vi "DunkFlips.vi"() -> ()   [LabVIEW 2015]
uses:
  <vilib>/eio/EIONode/EIONode.xnode
  <vilib>/rvi/eio/common/nirviEmuTemplateMethod_errors.vi
  <vilib>/rvi/DataTransferAndStorage/Container/XNode/niFpgaContainer.xnode
  <vilib>/rvi/LocalResourceManager/LocalResourceManager.xnode
  <vilib>/rvi/FIFO/Fifo_Resource/niFpgaFifoEmulationRefIn.vi
  <vilib>/rvi/DataTransferAndStorage/Container/Common/niFpgaContainerGetUniqueNameForEmu.vi
  <vilib>/rvi/DataTransferAndStorage/Container/Common/niFpgaContainerSetEmuInfo.vi
  <vilib>/rvi/eio/common/nirviEmuReportErrorAndStop.vi
  <vilib>/rvi/Analysis/measure/period/XNode/niFpgaAnalogPeriod.xnode
  <vilib>/rvi/Analysis/measure/period/templates/niFPGA Period Edge Direction.ctl
  <vilib>/rvi/Analysis/common/codeGenErrors/XNode/niFpgaXNodeCodeGenErrorHandle.vi
  <vilib>/rvi/Analysis/utilities/niFPGA Threshold Crossing Logic.vi
  <vilib>/Platform/TimedLoop/XDataNode/XDataNode.xnode
  <vilib>/Platform/TimedLoop/XDataNode/timing_clust.ctl
  <vilib>/Platform/TimedLoop/XDataNode/XDNodeRunTimeDep.lvlib
  <vilib>/Platform/TimedLoop/XDataNode/wakeup.ctl
  <vilib>/Platform/TimedLoop/XDataNode/nitl_modes.ctl
  <vilib>/rvi/FXPMathLib/basic elements/FxpDiscreteDelay/XNode/nifxpmath_DiscreteDelay.xnode
  <vilib>/rvi/interface/RandomDataEmulation/nirviRandomDataFpgaReadWriteTemplate.vi
  <vilib>/rvi/Analysis/measure/butterworth/XNode/niFpgaButterworthFilter.xnode
panel:
  in  "High Pass":bool
  in  "Low Pass":bool
  in  "Hysteresis 4":fxp<+,8,7> format="%#_13g"
  in  "Hysteresis 3":fxp<+,8,7> format="%#_13g"
  in  "Hysteresis 2":fxp<+,8,7> format="%#_13g"
  out "Actual Sample Period Process (ticks)":u32=80
  in  "Min signal time gap (samples)":u32=1000000
  in  "Min Amplitude 1":fxp<+,16,8>
  out "Output 1":i32
  out "AI0":sgl(slide) scale=-10.0..10.0
  in  "Min Amplitude 2":fxp<+,16,8>
  out "Output 2":i32
  out "AI1":sgl(slide) scale=-10.0..10.0
  in  "Min Amplitude 3":fxp<+,16,8>
  out "Output 3":i32
  out "AI2":sgl(slide) scale=-10.0..10.0
  out "Output 4":i32
  in  "Max Period (samples)":fxp<+,16,16>=65535.0 format="%#_13g"
  in  "Min Period (samples)":fxp<+,16,16> format="%#_13g"
  in  "Hysteresis 1":fxp<+,8,7> format="%#_13g"
  in  "Min Amplitude 4":fxp<+,16,8>
  out "AI3":sgl(slide)=8.326673e-17 scale=-10.0..10.0
  in  "Requested Sample Period (ticks)":u32=80
  out "Invalid Period":bool
  out "Actual Sample Period Wave (ticks)":u32=80
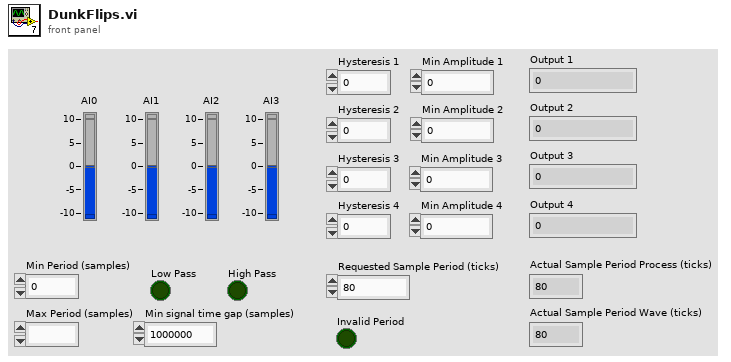
[diagram p1: front panel]
types:
  T1 = typedef "XDNodeRunTimeDep.lvlib/timing_clust.ctl" = cluster{"Expected End [f-1]":u64, "Actual End [f-1]":u64, "Finished Late? [f-1]":bool, "Expected End [i-1]":u64, "Actual End [i-1]":u64, "Finished Late? [i-1]":bool, "Expected Start [i]":u64, "Actual Start [i]":u64, "Expected Start [f]":u64, "Actual Start [f]":u64, "Source Name":string, "Structure Name":string, "Period":i64, "Deadline":i64, "Offset":i64, "Start":i64, "Priority":i32, "Timeout":i32, "Mode":T2, "Wakeup Reason":T3, "Error":errorcluster, "Source Type":string, "Secondary Source Type":string, "Global End Time":u64, "Global Start Time":u64, "Frame Duration":u64, "Iteration Duration":u64, "Assigned CPU":i32, "I/O Scan Engine Mode":u32}
  T2 = typedef "XDNodeRunTimeDep.lvlib/nitl_modes.ctl" = enum32{"No Change", "Process missed periods, maintain original phase", "Discard missed periods, maintain original phase", "Process missed periods, ignore original phase", "Discard missed periods, ignore original phase"}
  T3 = typedef "XDNodeRunTimeDep.lvlib/wakeup.ctl" = enum32{"Normal", "Aborted", "Asynchronous wakeup", "Timing source error", "Timed loop error", "Timeout"}
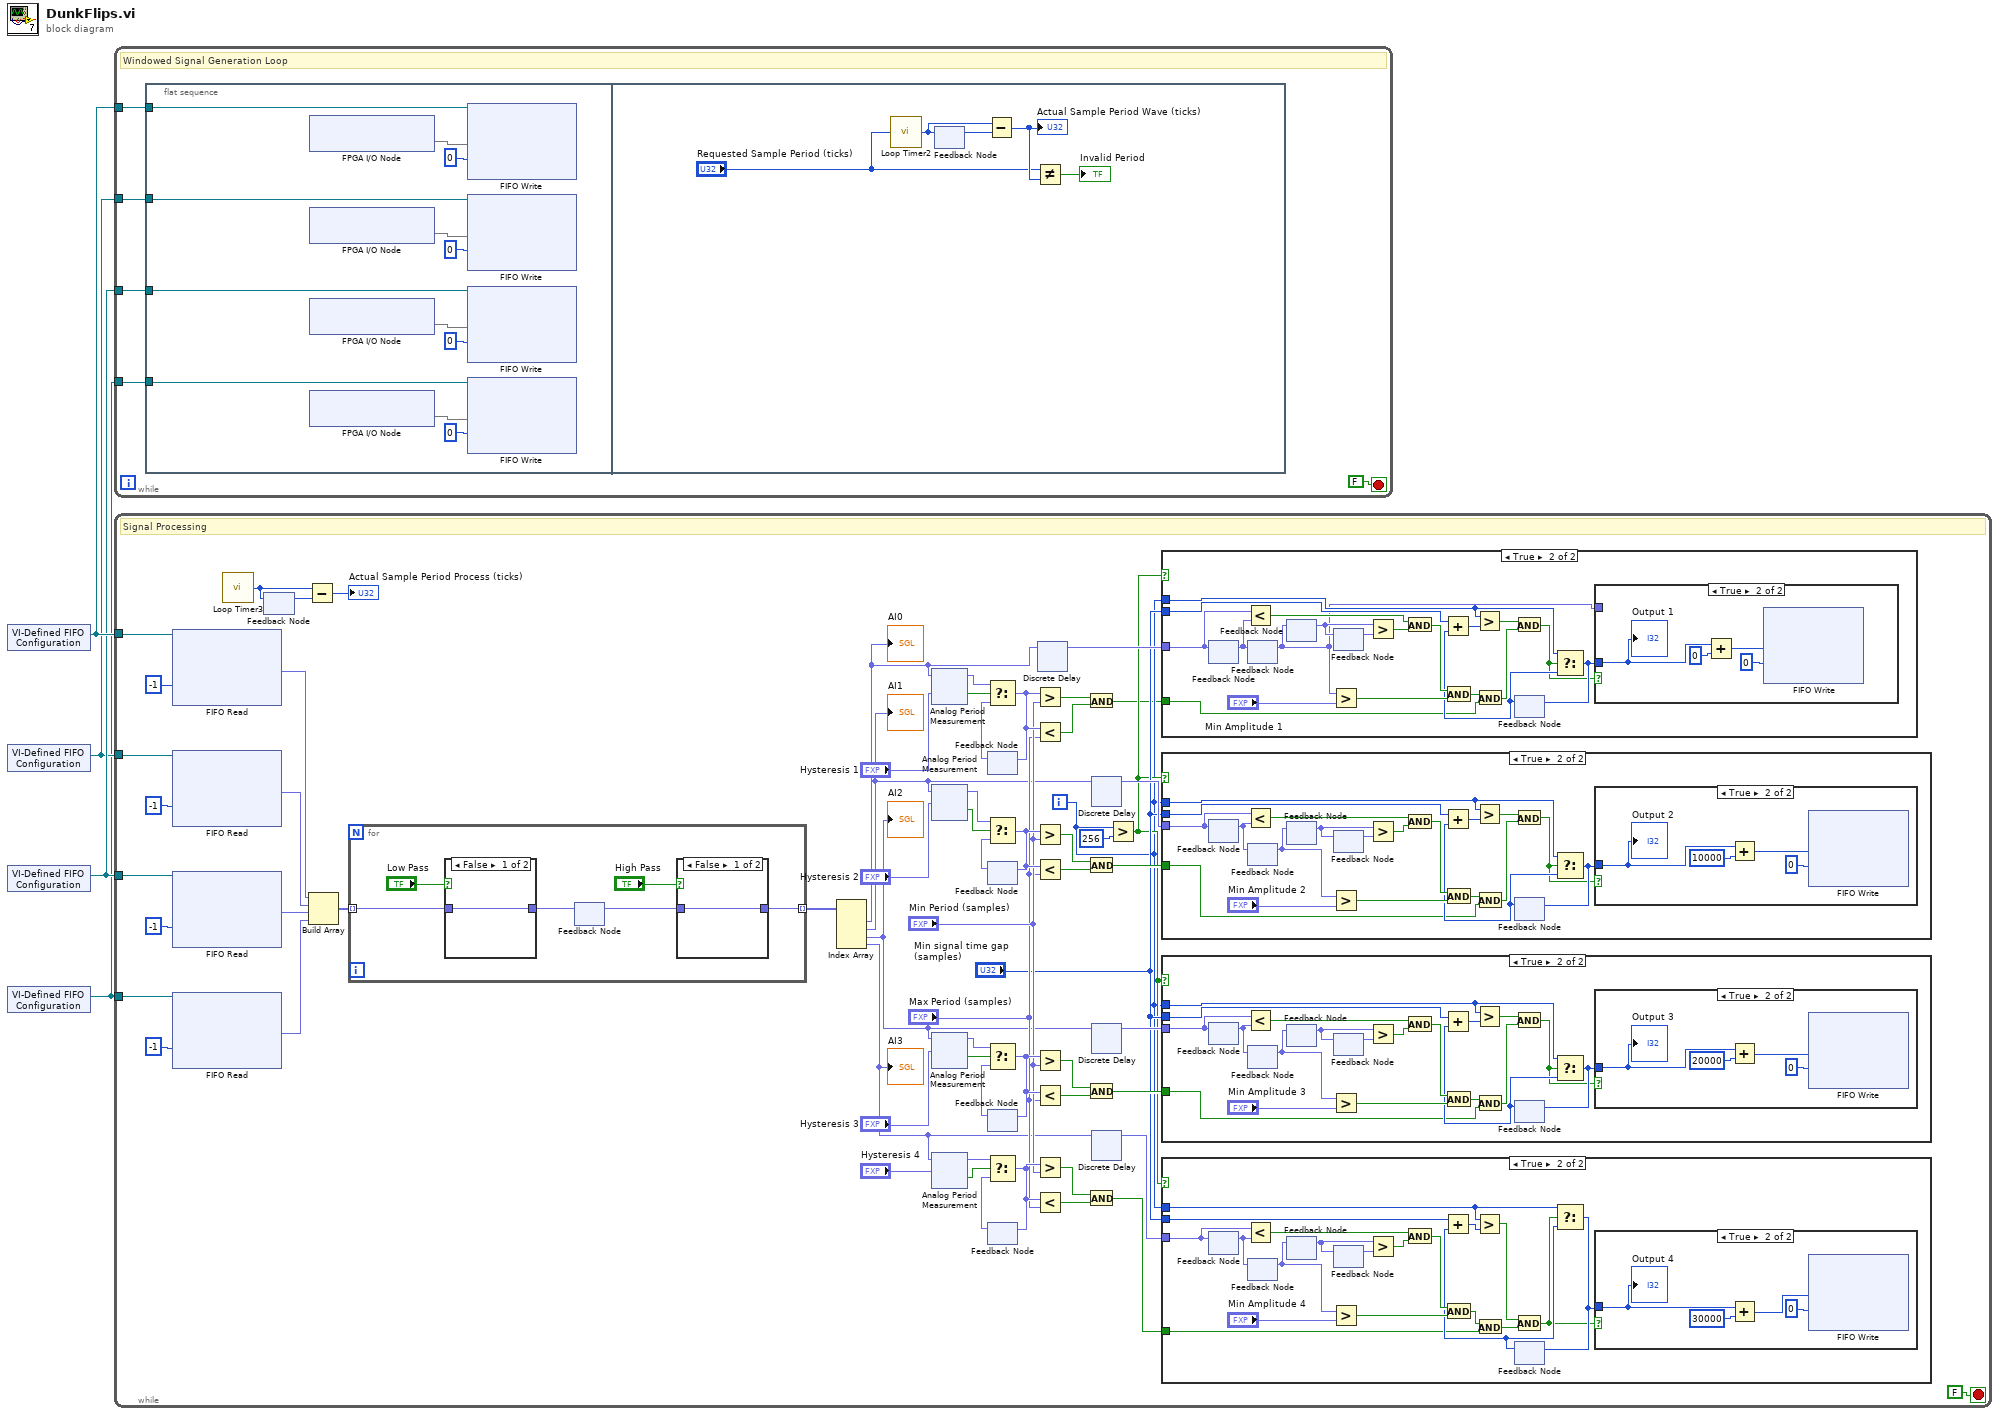
[diagram p0: block diagram]
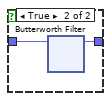
[diagram p2: hidden frame]
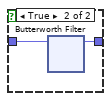
[diagram p3: hidden frame]
diagram:
  n1 = xnode "VI-Defined FIFO Configuration"() -> ("FIFO Out"=w4:refnum<k21>)
  n2 = xnode "VI-Defined FIFO Configuration"() -> ("FIFO Out"=w2:refnum<k21>)
  n3 = xnode "VI-Defined FIFO Configuration"() -> ("FIFO Out"=w3:refnum<k21>)
  n4 = xnode "VI-Defined FIFO Configuration"() -> ("FIFO Out"=w1:refnum<k21>)
  n5 = while {
    tunnel: w4 -> [w9]
    tunnel: w2 -> [w7]
    tunnel: w3 -> [w6]
    tunnel: w1 -> [w5]
    stop <- FALSE stop-if-true
    # "Windowed Signal Generation Loop"
    n6 = flat-sequence {
      tunnel: w9 -> [w16]
      tunnel: w7 -> [w15]
      tunnel: w6 -> [w14]
      tunnel: w5 -> [w17]
      frame #0 {
        n7 = xnode "FPGA I/O Node"() -> ("Connector0/AI0"=w13)  [unwired: 1 in, 1 out]
        n8 = xnode "FPGA I/O Node"() -> ("Connector0/AI1"=w10)  [unwired: 1 in, 1 out]
        n9 = xnode "FPGA I/O Node"() -> ("Connector0/AI2"=w11)  [unwired: 1 in, 1 out]
        n10 = xnode "FPGA I/O Node"() -> ("Connector0/AI3"=w12)  [unwired: 1 in, 1 out]
        n11 = xnode ("FIFO Write")("Element"=w13, "Timeout"=0, "FIFO In"=w16) -> ()  [unwired: 2 out]
        n12 = xnode ("FIFO Write")("Element"=w10, "Timeout"=0, "FIFO In"=w15) -> ()  [unwired: 2 out]
        n13 = xnode ("FIFO Write")("Element"=w11, "Timeout"=0, "FIFO In"=w14) -> ()  [unwired: 2 out]
        n14 = xnode ("FIFO Write")("Element"=w12, "Timeout"=0, "FIFO In"=w17) -> ()  [unwired: 2 out]
      }
      frame #1 {
        n15 = call "Loop Timer2"("Count(Ticks)"="Requested Sample Period (ticks)") -> ("Tick Count(Ticks)"=w22:u32)
        n16 = feedback #1() -> (w23:u32)  [unwired: 1 in]
        n17 = feedback-in #1(w22) -> ()
        n18 = Subtract(x=w22, y=w23) -> (x-y=w26:u32)
        "Actual Sample Period Wave (ticks)" <- w26
        n19 = Not Equal?(x="Requested Sample Period (ticks)", y=w26) -> (x != y?=→"Invalid Period":bool)
      }
    }
  }
  n20 = while {
    tunnel: w4 -> [w60]
    tunnel: w2 -> [w61]
    tunnel: w3 -> [w59]
    tunnel: w1 -> [w81]
    i -> [w50]
    stop <- FALSE stop-if-true
    # "Signal Processing"
    n21 = xnode ("FIFO Read")("Timeout"=i16 -1, "FIFO In"=w60) -> ("Element"=w30:fxp<+/-,16,4>)  [unwired: 2 out]
    n22 = xnode ("FIFO Read")("Timeout"=i16 -1, "FIFO In"=w61) -> ("Element"=w29:fxp<+/-,16,4>)  [unwired: 2 out]
    n23 = xnode ("FIFO Read")("Timeout"=i16 -1, "FIFO In"=w59) -> ("Element"=w28:fxp<+/-,16,4>)  [unwired: 2 out]
    n24 = xnode ("FIFO Read")("Timeout"=i16 -1, "FIFO In"=w81) -> ("Element"=w27:fxp<+/-,16,4>)  [unwired: 2 out]
    n25 = call "Loop Timer3"() -> ("Tick Count(Ticks)"=w51:u32)  [unwired: 1 in]
    n26 = feedback #2() -> (w52:u32)  [unwired: 1 in]
    n27 = feedback-in #2(w51) -> ()
    n28 = Subtract(x=w51, y=w52) -> (x-y=→"Actual Sample Period Process (ticks)":u32)
    n29 = Build Array(w30, w29, w28, w27) -> (w36:fxp<+/-,16,4>[])
    n30 = for {
      tunnel: w36 -> [w93] mode=indexing
      tunnel: [w94] -> w35 mode=indexing
      n31 = case shown="False" "Low Pass" {
        tunnel: [w109 w111] -> w96
        tunnel: w93 -> [w109 w110]
        frame False {
        }
        frame True {
          n32 = xnode "Butterworth Filter"("input data"=w110) -> ("output data"=w111:fxp<+/-,20,8>)  [unwired: 2 in, 1 out]
        }
      }
      n33 = feedback #3() -> (w95:fxp<+/-,20,8>)  [unwired: 1 in]
      n34 = feedback-in #3(w96) -> ()
      n35 = case shown="False" "High Pass" {
        tunnel: w95 -> [w97 w99]
        tunnel: [w97 w98] -> w94
        frame False {
        }
        frame True {
          n36 = xnode "Butterworth Filter"("input data"=w99) -> ("output data"=w98:fxp<+/-,20,12>)  [unwired: 2 in, 1 out]
        }
      }
    }
    n37 = Index Array(array=w35) -> (element #1=w34:fxp<+/-,24,12>, element #2=w33:fxp<+/-,24,12>, element #3=w32:fxp<+/-,24,12>, element #4=w31:fxp<+/-,24,12>)  [unwired: 4 in]
    "AI3" <- w31
    "AI2" <- w32
    "AI1" <- w33
    "AI0" <- w34
    n38 = xnode "Analog Period Measurement"("input data"=w34, "direction"="Hysteresis 1") -> ("period (samples)"=w48:fxp<+,32,16>, "output valid"=w64:bool)  [unwired: 3 in, 2 out]
    n39 = xnode "Analog Period Measurement"("input data"=w33, "hysteresis"="Hysteresis 2") -> ("period (samples)"=w46:fxp<+,32,16>, "output valid"=w69:bool)  [unwired: 3 in, 2 out]
    n40 = xnode "Analog Period Measurement"("input data"=w32, "hysteresis"="Hysteresis 3") -> ("period (samples)"=w44:fxp<+,32,16>, "output valid"=w75:bool)  [unwired: 3 in, 2 out]
    n41 = xnode "Analog Period Measurement"("input data"=w31, "hysteresis"="Hysteresis 4") -> ("period (samples)"=w42:fxp<+,32,16>, "output valid"=w83:bool)  [unwired: 3 in, 2 out]
    n42 = feedback #4() -> (w47:fxp<+,32,16>)  [unwired: 1 in]
    n43 = Select(t=w48, s=w64, f=w47) -> (s? t:f=w66:fxp<+,32,16>)
    n44 = feedback-in #4(w66) -> ()
    n45 = feedback #5() -> (w45:fxp<+,32,16>)  [unwired: 1 in]
    n46 = Select(t=w46, s=w69, f=w45) -> (s? t:f=w71:fxp<+,32,16>)
    n47 = feedback-in #5(w71) -> ()
    n48 = feedback #6() -> (w43:fxp<+,32,16>)  [unwired: 1 in]
    n49 = Select(t=w44, s=w75, f=w43) -> (s? t:f=w77:fxp<+,32,16>)
    n50 = feedback-in #6(w77) -> ()
    n51 = feedback #7() -> (w41:fxp<+,32,16>)  [unwired: 1 in]
    n52 = Select(t=w42, s=w83, f=w41) -> (s? t:f=w86:fxp<+,32,16>)
    n53 = feedback-in #7(w86) -> ()
    n54 = Greater?(x=w66, y="Min Period (samples)") -> (0:w68:bool)
    n55 = Less?(x=w66, y="Max Period (samples)") -> (x < y?=w67:bool)
    n56 = Greater?(x=w71, y="Min Period (samples)") -> (0:w73:bool)
    n57 = Less?(x=w71, y="Max Period (samples)") -> (x < y?=w72:bool)
    n58 = Greater?(x=w77, y="Min Period (samples)") -> (0:w79:bool)
    n59 = Less?(x=w77, y="Max Period (samples)") -> (x < y?=w78:bool)
    n60 = Greater?(x=w86, y="Min Period (samples)") -> (0:w88:bool)
    n61 = Less?(x=w86, y="Max Period (samples)") -> (x < y?=w87:bool)
    n62 = xnode ("Discrete Delay")("D"=w34) -> ("Q"=w65:fxp<+/-,24,12>)
    n63 = And(x=w68, y=w67) -> (x .and. y?=w49:bool)
    n64 = And(x=w73, y=w72) -> (x .and. y?=w74:bool)
    n65 = And(x=w79, y=w78) -> (x .and. y?=w80:bool)
    n66 = And(x=w88, y=w87) -> (x .and. y?=w89:bool)
    n67 = xnode ("Discrete Delay")("D"=w33) -> ("Q"=w70:fxp<+/-,24,12>)
    n68 = xnode ("Discrete Delay")("D"=w32) -> ("Q"=w76:fxp<+/-,24,12>)
    n69 = xnode ("Discrete Delay")("D"=w31) -> ("Q"=w84:fxp<+/-,24,12>)
    n70 = Greater?(x=w50, y=i16 256) -> (0:w57:bool)
    n71 = case shown="True" w57 {
      tunnel: w50 -> [_ w134]
      tunnel: w65 -> [_ w130]
      tunnel: w49 -> [_ w126]
      tunnel: "Min signal time gap (samples)" -> [_ w125]
      frame False {
      }
      frame True {
        n72 = feedback #8() -> (w138:fxp<+/-,24,12>)  [unwired: 1 in]
        n73 = feedback-in #8(w130) -> ()
        n74 = Less?(x=w130, y=w138) -> (x < y?=w122:bool)
        n75 = feedback #9() -> (w121:fxp<+/-,24,12>)  [unwired: 1 in]
        n76 = feedback-in #9(w138) -> ()
        n77 = feedback #10() -> (w139:fxp<+/-,24,12>)  [unwired: 1 in]
        n78 = feedback-in #10(w121) -> ()
        n79 = Greater?(x=w121, y="Min Amplitude 1") -> (0:w133:bool)
        n80 = feedback #11() -> (w140:fxp<+/-,24,12>)  [unwired: 1 in]
        n81 = feedback-in #11(w139) -> ()
        n82 = Greater?(x=w139, y=w140) -> (0:w123:bool)
        n83 = And(x=w122, y=w123) -> (x .and. y?=w135:bool)
        n84 = And(x=w135, y=w133) -> (x .and. y?=w128:bool)
        n85 = And(x=w128, y=w126) -> (x .and. y?=w127:bool)
        n86 = feedback #12() -> (w131:i32)  [unwired: 1 in]
        n87 = Add(x=w125, y=w131) -> (x+y=w137:u32)
        n88 = Greater?(x=w134, y=w137) -> (0:w124:bool)
        n89 = And(x=w124, y=w127) -> (x .and. y?=w129:bool)
        n90 = Select(t=w134, s=w129, f=w131) -> (s? t:f=w132:i32)
        n91 = feedback-in #12(w132) -> ()
        n92 = case shown="True" w129 {
          tunnel: w132 -> [_ w142]
          tunnel: w121 -> [_ _]
          frame False {
          }
          frame True {
            n93 = Add(x=w142, y=i16 0) -> (x+y=w141:i32)
            n94 = xnode ("FIFO Write")("Element"=w141, "Timeout"=i16 0) -> ()  [unwired: 1 in, 2 out]
            "Output 1" <- w142
          }
        }
      }
    }
    n95 = case shown="True" w57 {
      tunnel: w50 -> [_ w274]
      tunnel: w70 -> [_ w269]
      tunnel: w74 -> [_ w265]
      tunnel: "Min signal time gap (samples)" -> [_ w264]
      frame False {
      }
      frame True {
        n96 = feedback #13() -> (w279:fxp<+/-,24,12>)  [unwired: 1 in]
        n97 = feedback-in #13(w269) -> ()
        n98 = Less?(x=w269, y=w279) -> (x < y?=w263:bool)
        n99 = feedback #14() -> (w277:fxp<+/-,24,12>)  [unwired: 1 in]
        n100 = feedback-in #14(w279) -> ()
        n101 = feedback #15() -> (w280:fxp<+/-,24,12>)  [unwired: 1 in]
        n102 = feedback-in #15(w277) -> ()
        n103 = Greater?(x=w277, y="Min Amplitude 2") -> (0:w272:bool)
        n104 = feedback #16() -> (w281:fxp<+/-,24,12>)  [unwired: 1 in]
        n105 = feedback-in #16(w280) -> ()
        n106 = Greater?(x=w280, y=w281) -> (0:w262:bool)
        n107 = And(x=w263, y=w262) -> (x .and. y?=w275:bool)
        n108 = And(x=w275, y=w272) -> (x .and. y?=w267:bool)
        n109 = And(x=w267, y=w265) -> (x .and. y?=w266:bool)
        n110 = feedback #17() -> (w270:i32)  [unwired: 1 in]
        n111 = Add(x=w264, y=w270) -> (x+y=w278:u32)
        n112 = Greater?(x=w274, y=w278) -> (0:w273:bool)
        n113 = And(x=w273, y=w266) -> (x .and. y?=w268:bool)
        n114 = Select(t=w274, s=w268, f=w270) -> (s? t:f=w271:i32)
        n115 = feedback-in #17(w271) -> ()
        n116 = case shown="True" w268 {
          tunnel: w271 -> [_ w283]
          frame False {
          }
          frame True {
            n117 = Add(x=w283, y=i16 10000) -> (x+y=w282:i32)
            n118 = xnode ("FIFO Write")("Element"=w282, "Timeout"=i16 0) -> ()  [unwired: 1 in, 2 out]
            "Output 2" <- w283
          }
        }
      }
    }
    n119 = case shown="True" w57 {
      tunnel: w50 -> [_ w415]
      tunnel: w76 -> [_ w410]
      tunnel: w80 -> [_ w406]
      tunnel: "Min signal time gap (samples)" -> [_ w405]
      frame False {
      }
      frame True {
        n120 = feedback #18() -> (w420:fxp<+/-,24,12>)  [unwired: 1 in]
        n121 = feedback-in #18(w410) -> ()
        n122 = Less?(x=w410, y=w420) -> (x < y?=w403:bool)
        n123 = feedback #19() -> (w418:fxp<+/-,24,12>)  [unwired: 1 in]
        n124 = feedback-in #19(w420) -> ()
        n125 = feedback #20() -> (w421:fxp<+/-,24,12>)  [unwired: 1 in]
        n126 = feedback-in #20(w418) -> ()
        n127 = Greater?(x=w418, y="Min Amplitude 3") -> (0:w413:bool)
        n128 = feedback #21() -> (w422:fxp<+/-,24,12>)  [unwired: 1 in]
        n129 = feedback-in #21(w421) -> ()
        n130 = Greater?(x=w421, y=w422) -> (0:w404:bool)
        n131 = And(x=w403, y=w404) -> (x .and. y?=w416:bool)
        n132 = And(x=w416, y=w413) -> (x .and. y?=w408:bool)
        n133 = And(x=w408, y=w406) -> (x .and. y?=w407:bool)
        n134 = feedback #22() -> (w411:i32)  [unwired: 1 in]
        n135 = Add(x=w405, y=w411) -> (x+y=w419:u32)
        n136 = Greater?(x=w415, y=w419) -> (0:w414:bool)
        n137 = And(x=w414, y=w407) -> (x .and. y?=w409:bool)
        n138 = Select(t=w415, s=w409, f=w411) -> (s? t:f=w412:i32)
        n139 = feedback-in #22(w412) -> ()
        n140 = case shown="True" w409 {
          tunnel: w412 -> [_ w424]
          frame False {
          }
          frame True {
            n141 = Add(x=w424, y=i16 20000) -> (x+y=w423:i32)
            n142 = xnode ("FIFO Write")("Element"=w423, "Timeout"=i16 0) -> ()  [unwired: 1 in, 2 out]
            "Output 3" <- w424
          }
        }
      }
    }
    n143 = case shown="True" w57 {
      tunnel: w50 -> [_ w556]
      tunnel: w84 -> [_ w551]
      tunnel: w89 -> [_ w547]
      tunnel: "Min signal time gap (samples)" -> [_ w546]
      frame False {
      }
      frame True {
        n144 = feedback #23() -> (w561:fxp<+/-,24,12>)  [unwired: 1 in]
        n145 = feedback-in #23(w551) -> ()
        n146 = Less?(x=w551, y=w561) -> (x < y?=w544:bool)
        n147 = feedback #24() -> (w559:fxp<+/-,24,12>)  [unwired: 1 in]
        n148 = feedback-in #24(w561) -> ()
        n149 = feedback #25() -> (w562:fxp<+/-,24,12>)  [unwired: 1 in]
        n150 = feedback-in #25(w559) -> ()
        n151 = Greater?(x=w559, y="Min Amplitude 4") -> (0:w554:bool)
        n152 = feedback #26() -> (w563:fxp<+/-,24,12>)  [unwired: 1 in]
        n153 = feedback-in #26(w562) -> ()
        n154 = Greater?(x=w562, y=w563) -> (0:w545:bool)
        n155 = And(x=w544, y=w545) -> (x .and. y?=w557:bool)
        n156 = And(x=w557, y=w554) -> (x .and. y?=w549:bool)
        n157 = And(x=w549, y=w547) -> (x .and. y?=w548:bool)
        n158 = feedback #27() -> (w552:i32)  [unwired: 1 in]
        n159 = Add(x=w546, y=w552) -> (x+y=w560:u32)
        n160 = Greater?(x=w556, y=w560) -> (0:w555:bool)
        n161 = And(x=w555, y=w548) -> (x .and. y?=w550:bool)
        n162 = Select(t=w556, s=w550, f=w552) -> (s? t:f=w553:i32)
        n163 = feedback-in #27(w553) -> ()
        n164 = case shown="True" w550 {
          tunnel: w553 -> [_ w565]
          frame False {
          }
          frame True {
            n165 = Add(x=w565, y=i16 30000) -> (x+y=w564:i32)
            n166 = xnode ("FIFO Write")("Element"=w564, "Timeout"=i16 0) -> ()  [unwired: 1 in, 2 out]
            "Output 4" <- w565
          }
        }
      }
    }
  }
